vi "Test NI DAQ API.vi"() -> ()   [LabVIEW 2020]
doc: "NI DAQ API Tester."
uses:
  Support/Task list.ctl
  AI config parameters--cluster.ctl
  <vilib>/Utility/error.llb/DialogType.ctl
  Support/Continuous aquisition params.ctl
  NI DAQ.lvlib
  <resource>/objmgr/daqmx.rc
panel:
  in  "Delete task":bool
  out "Digital data":bool[](array[boolean])
  out "Analog data":dbl[](array[numeric])
  in  "Stop continuous acquisition":bool
  in  "N samples":i32
  in  "Acquisition type":enum16{"Single", "Multiple"}(ring)=enum."Multiple"
  in  "Start continous acquisition":bool
  out "DevSerialNum":u32
  out "Connection valid?":bool
  in  "Validate connection":bool
  in  "Sleep HL":bool
  in  "Task list":T1=enum."DO task"
  in  "Timeout":i32=100
  in  "Wake up HL":bool
  in  "Task list 2":T1 caption="Task to get"
  out "DAQmx Task":refnum<k21>
  in  "Get task ref":bool
  in  "Task to stop/delete":T2(ring)
  in  "Tab Control":enum32{"DO", "DI", "AI", "AO"}(tab)
  in  "Create DO task":bool
  in  "Write DO":bool
  in  "Samples":enum16{"Single", "Multiple"}(ring)
  in  "Data":bool[](array[boolean])
  in  "Create DI channel":bool
  in  "Samples 2":enum16{"Single", "Multiple"}(ring) caption="Samples"
  in  "Read DI":bool
  out "Data read":bool[](array[boolean])
  in  "Create AI channel":bool
  in  "Config params":T3={"Terminal configuration"=-1, "min value"=-5.0, "max value"=5.0} {"max value" format="%0.2f"; "min value" format="%0.2f"; "Terminal configuration" items=["Default"=-1, "RSE"=10083, "NRSE"=10078, "Differential"=10106, "Pseudodifferential"=12529]}
  in  "Read AI":bool
  in  "Samples 3":enum16{"Single", "Multiple"}(ring) caption="Samples"
  out "AI Data":dbl[](array[numeric])
  in  "Create AO channel":bool
  in  "Config params 2":T3={"Terminal configuration"=-1, "min value"=-5.0, "max value"=5.0} caption="Config params" {"max value" format="%0.2f"; "min value" format="%0.2f"; "Terminal configuration" items=["Default"=-1, "RSE"=10083, "NRSE"=10078, "Differential"=10106, "Pseudodifferential"=12529]}
  in  "Write AO":bool
  in  "Value(s)":dbl[](array[numeric])
  in  "Samples 4":enum16{"Single", "Multiple"}(ring) caption="Samples"
  in  "Stop task":bool
  in  "Start task":bool
  in  "Channel name":string
  in  "Physical channel(s)":string
  out "Available channels":i32(listbox)
  in  "Get channel list":bool
  in  "Set device ID":bool
  in  "Avilable devices":u16(ring) items=["Dev1"]
  in  "Show Diagram on Init":bool
  in  "Run as Singleton?":bool
  in  "Show Block Diagram":bool
  in  "Refresh Modules":bool
  out "Active Modules":string[](array[string])
  in  "Stop Module":bool
  in  "Select Module":i32(ring)=-1 caption="Select Module\nTo send Request to" items=["All"=-1]
  in  "Run New Module":bool
  in  "Hide Module Panel":bool
  in  "Show Module Panel":bool
  out "Status":string
  # "This VI tests the API for the Module."
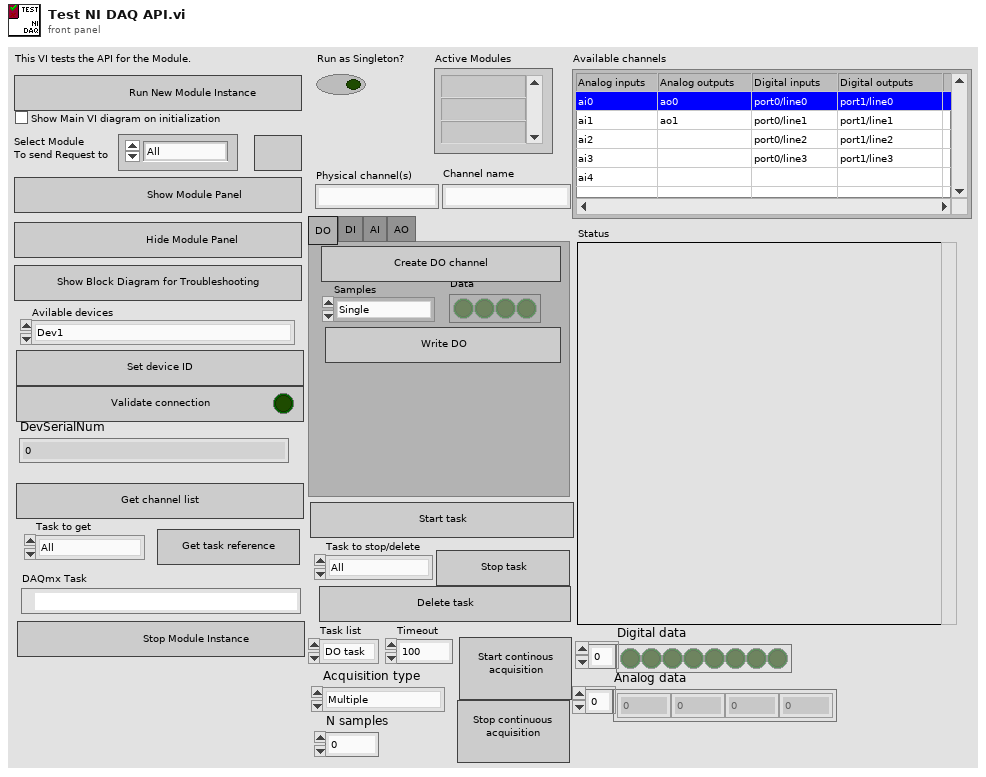
[diagram p1: front panel]
types:
  T1 = typedef "NI DAQ.lvlib/Task list.ctl" = enum16{"All", "DO task", "DI task", "AO task", "AI task"}
  T2 = enum16{"All", "DO task", "DI task", "AO task", "AI task"}
  T3 = typedef "NI DAQ.lvlib/AI config parameters--cluster.ctl" = cluster{"Terminal configuration":i32, "min value":dbl, "max value":dbl}
  T4 = typedef "NI DAQ.lvlib/Broadcast Events--cluster.ctl" = cluster{"Module Did Init":refnum<user-event>, "Status Updated":refnum<user-event>, "Error Reported":refnum<user-event>, "Module Did Stop":refnum<user-event>, "Update Module Execution Status":refnum<user-event>, "Digital data acquired":refnum<user-event>, "Device connected":refnum<user-event>, "Connection failed":refnum<user-event>, "Analog data acquired":refnum<user-event>, "Tasks started":refnum<user-event>}
  T5 = typedef "NI DAQ.lvlib/Continuous aquisition params.ctl" = cluster{"Module ID":i32, "Task list":T1, "Timeout":i32, "Acq type":enum16{"Single", "Multiple"}, "Data in":variant, "DAQmx Task":refnum<k21>, "N samples":i32}
  T6 = typedef "DialogType.ctl" = u16
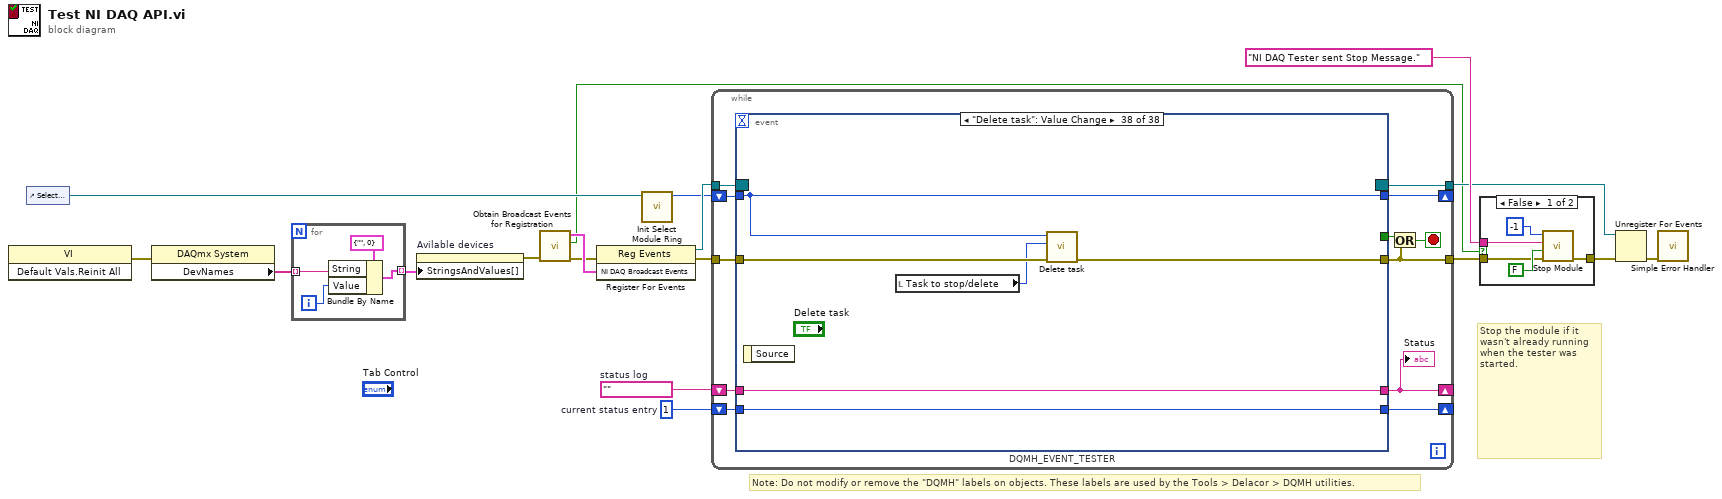
[diagram p0: block diagram]
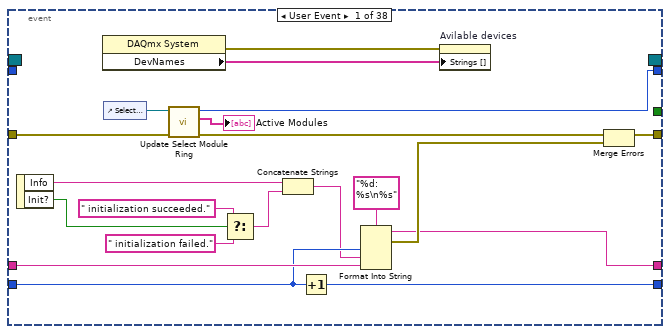
[diagram p3: hidden frame]
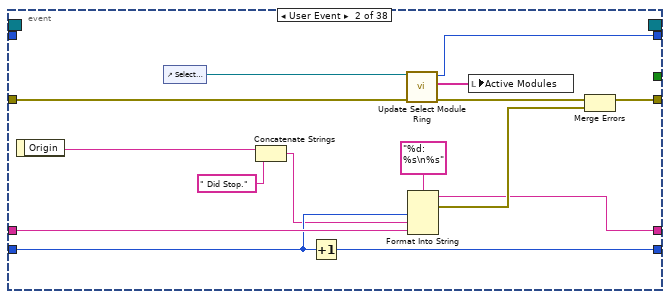
[diagram p4: hidden frame]
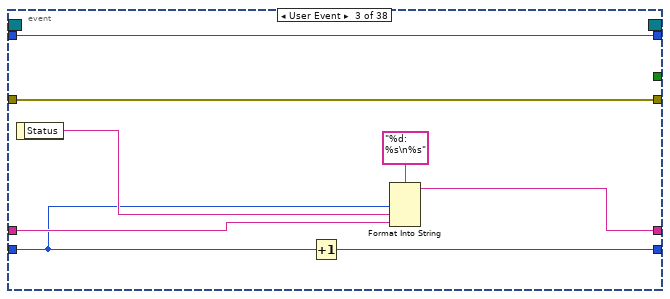
[diagram p5: hidden frame]
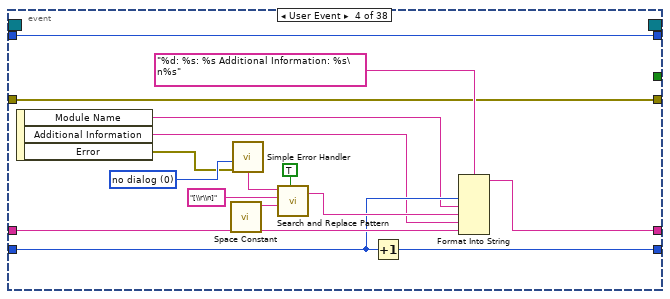
[diagram p6: hidden frame]
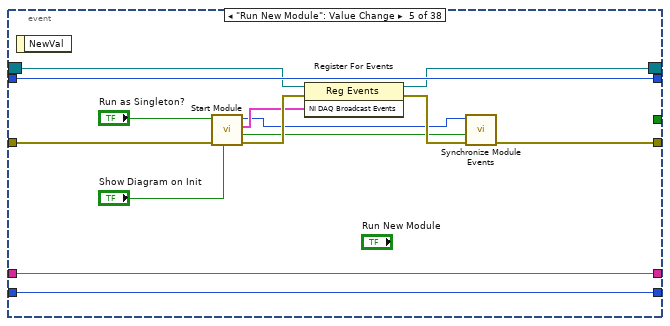
[diagram p7: hidden frame]
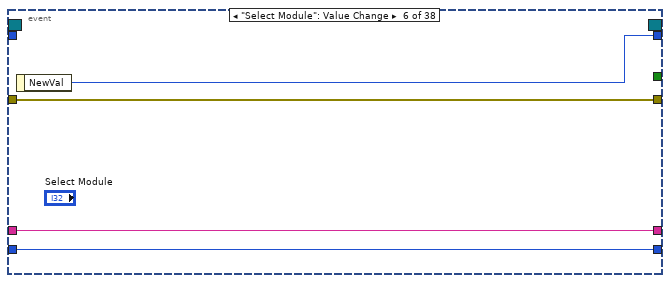
[diagram p8: hidden frame]
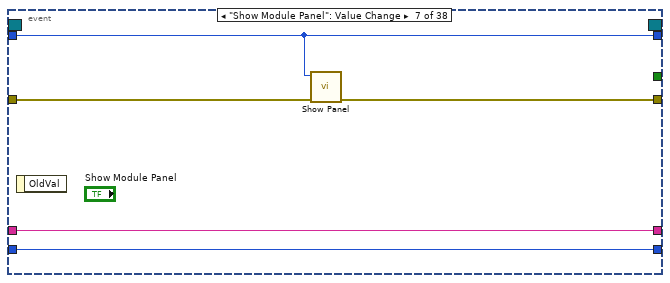
[diagram p9: hidden frame]
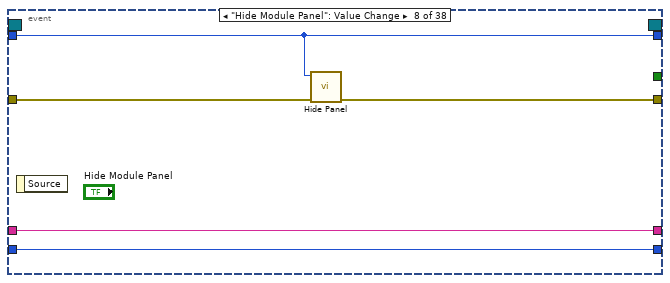
[diagram p10: hidden frame]
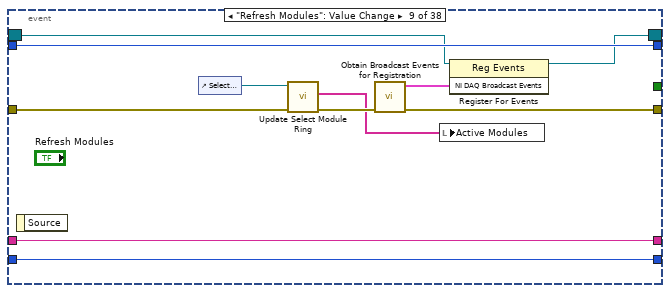
[diagram p11: hidden frame]
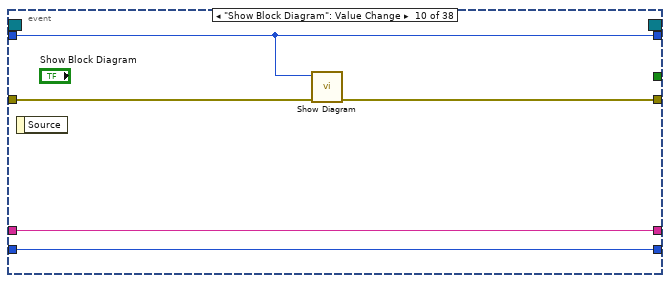
[diagram p12: hidden frame]
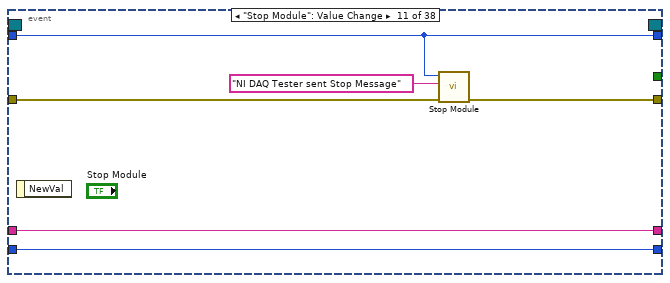
[diagram p13: hidden frame]
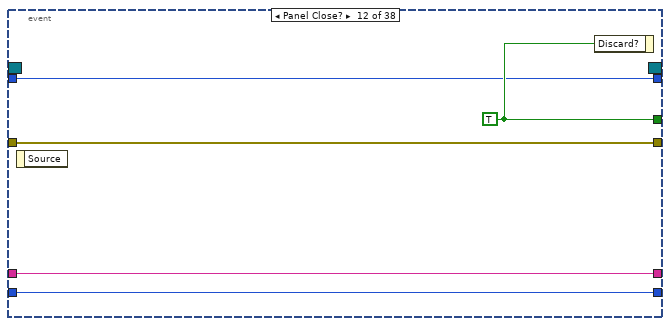
[diagram p14: hidden frame]
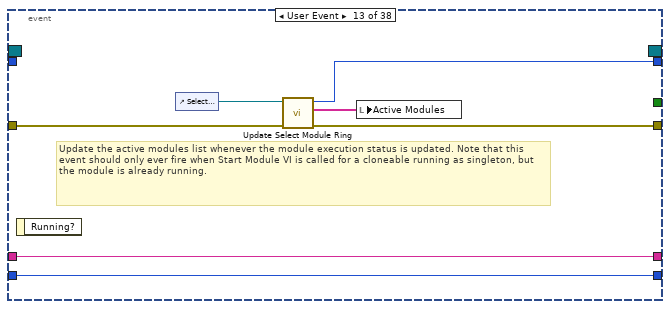
[diagram p15: hidden frame]
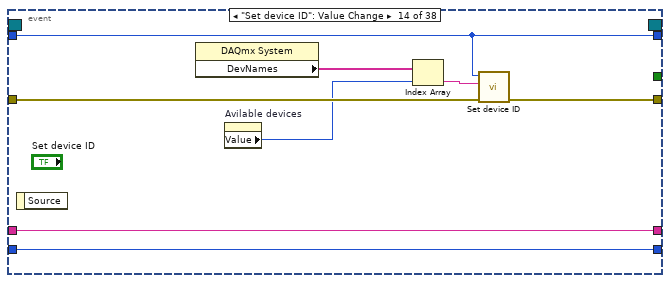
[diagram p16: hidden frame]
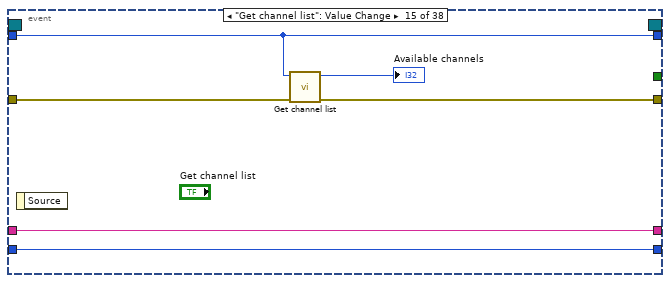
[diagram p17: hidden frame]
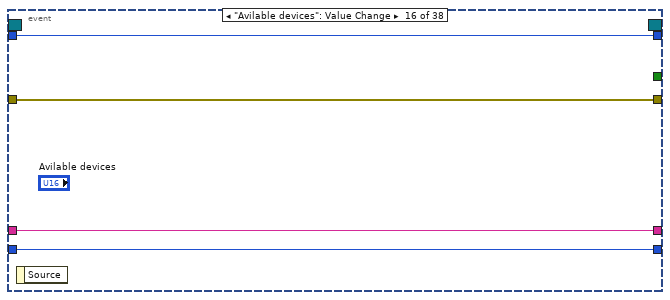
[diagram p18: hidden frame]
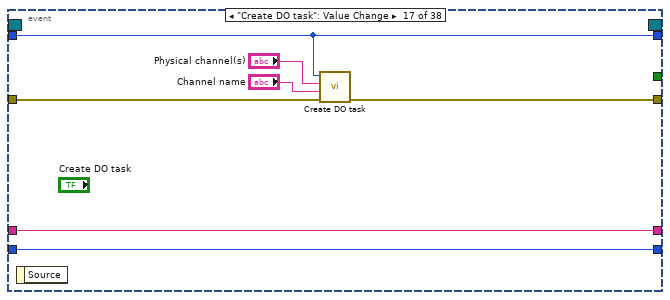
[diagram p19: hidden frame]
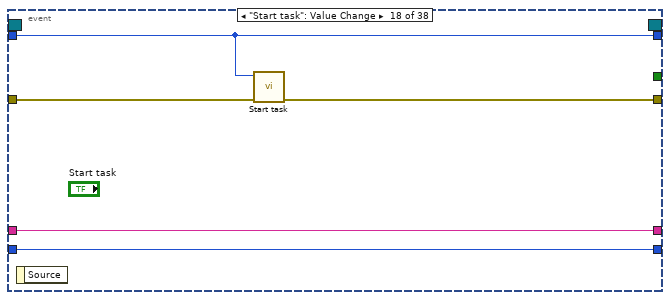
[diagram p20: hidden frame]
diagram:
  w15 = 1  # current status entry
  w16 = ""  # status log
  # "Stop the module if it wasn't already running when the tester was started."
  # "Note: Do not modify or remove the \"DQMH\" labels on objects. These labels are used by the Tools > Delacor > DQMH utilities."
  n1 = invoke class="VI" method="Default Vals.Reinit All"() -> (error out=w4:errorcluster)  [unwired: 3 in, 2 out]
  n2 = control-ref of="Select Module"() -> (w13:refnum<vi>)
  n3 = property class="DAQmx System"(error in=w4) -> ("DevNames"=w3:tag[])  [unwired: 1 in, 2 out]
  n4 = for {
    tunnel: w3 -> [w21] mode=indexing
    tunnel: [w19] -> w2 mode=indexing
    i -> [w20]
    n5 = Bundle By Name(cluster=cluster{"String":string, "Value":u16} {"String"="", "Value"=0} ("Cluster"), "String"=w21, "Value"=w20) -> (w19:cluster{"String":string, "Value":u16})
  }
  n6 = property on="Avilable devices" class="Ring (strict)"("StringsAndValues[]"=w2) -> (error out=w1:errorcluster)  [unwired: 2 in, 1 out]
  n7 = call "Obtain Broadcast Events for Registration.vi"("error in"=w1) -> ("error out"=w8:errorcluster, "Already running?"=w7:bool, "NI DAQ Broadcast Events"=w12:T4)  [unwired: 8 in]
  n8 = register-events(error in=w8, w12) -> (reference out=w18:refnum<event-registration>, error out=w11:errorcluster)  [unwired: 1 in]
  n9 = call "Init Select Module Ring.vi"("Select Module Ring Ref"=w13) -> ("Value for All Modules"=w14:i32)  [unwired: 8 in, 2 out]
  n10 = while {
    tunnel: w18 -> [w34]
    tunnel: [w23] -> w6
    tunnel: w11 -> [w32]
    shift-right: [w28] -> _
    shift-left: w16 -> [w30]
    shift-right: [w29] -> _
    shift-left: w15 -> [w31]
    shift-right: [w25] -> _
    shift-left: w14 -> [w26]
    tunnel: [w24] -> w9
    stop <- w27 stop-if-true
    n11 = event "DQMH_EVENT_TESTER" shown="[37] \"Delete task\": Value Change" {
      selector: w34 -> [_ _ _ _ w101 _ _ _ w127 _ _ _ _ _ _ _ _ _ _ _ _ _ _ _ _ _ _ _ _ _ _ _ _ _ _ _ _ _]
      dyn-events: [_ _ _ _ w100 _ _ _ w126 _ _ _ _ _ _ _ _ _ _ _ _ _ _ _ _ _ _ _ _ _ _ _ _ _ _ _ _ _] -> w24
      timeout: _ -> [_ _ _ _ _ _ _ _ _ _ _ _ _ _ _ _ _ _ _ _ _ _ _ _ _ _ _ _ _ _ _ _ _ _ _ _ _ _]
      tunnel: [_ _ _ _ _ _ _ _ _ _ _ w148 _ _ _ _ _ _ _ _ _ _ _ _ _ _ _ _ _ _ _ _ _ _ _ _ _ _] -> w33
      tunnel: [w45 w61 w77 w81 w99 w111 w115 w120 w123 w134 w139 w147 w151 w160 w166 w173 w177 w182 w188 w195 w202 w209 w216 w230 w234 w248 w253 w260 w268 w275 w281 w295 w306 w312 w317 w331 w341 w343] -> w23
      tunnel: w32 -> [w46 w63 w77 w81 w102 w111 w116 w121 w128 w137 w140 w147 w152 w163 w169 w173 w180 w185 w191 w198 w205 w212 w219 w229 w237 w248 w256 w263 w271 w278 w284 w295 w306 w315 w320 w331 w341 w347]
      tunnel: w31 -> [w51 w66 w70 w84 w104 w109 w113 w118 w131 w135 w142 w145 w154 w161 w167 w171 w178 w183 w189 w196 w203 w210 w217 w231 w235 w244 w254 w261 w269 w276 w282 w291 w302 w313 w318 w327 w337 w345]
      tunnel: w30 -> [w52 w67 w73 w85 w105 w110 w114 w119 w132 w136 w143 w146 w155 w162 w168 w172 w179 w184 w190 w197 w204 w211 w218 w232 w236 w246 w255 w262 w270 w277 w283 w293 w304 w314 w319 w329 w339 w346]
      tunnel: [w49 w64 w74 w83 w105 w110 w114 w119 w132 w136 w143 w146 w155 w162 w168 w172 w179 w184 w190 w197 w204 w211 w218 w232 w236 w245 w255 w262 w270 w277 w283 w292 w303 w314 w319 w328 w338 w346] -> w28
      tunnel: [w50 w65 w76 w82 w104 w109 w113 w118 w131 w135 w142 w145 w154 w161 w167 w171 w178 w183 w189 w196 w203 w210 w217 w231 w235 w243 w254 w261 w269 w276 w282 w290 w301 w313 w318 w326 w336 w345] -> w29
      tunnel: w26 -> [_ _ w71 w93 w103 _ w112 w117 w130 w133 w141 w144 _ w159 w165 w170 w176 w181 w187 w194 w201 w208 w215 w227 w233 w247 w252 w259 w267 w274 w280 w294 w305 w311 w316 w330 w340 w344]
      tunnel: [w37 w58 w71 w93 w103 w108 w112 w117 w130 w133 w141 w144 w150 w159 w165 w170 w176 w181 w187 w194 w201 w208 w215 w227 w233 w247 w252 w259 w267 w274 w280 w294 w305 w311 w316 w330 w340 w344] -> w25
      event User Event {
        n12 = event-data() -> ("Info"=w48:string, "Init?"=w40:bool)  [unwired: 1 in]
        n13 = property class="DAQmx System"() -> (error out=w36:errorcluster, "DevNames"=w35:tag[])  [unwired: 2 in, 1 out]
        n14 = control-ref of="Select Module"() -> (w44:refnum<vi>)
        n15 = call "Update Select Module Ring.vi"("error in (no error)"=w46, "Select Module Ring Ref"=w44) -> ("error out"=w38:errorcluster, "Active Modules (Array)"=→"Active Modules":string[], "New Module Ring Value"=w37:i32)  [unwired: 7 in]
        n16 = Select(t=" initialization succeeded.", s=w40, f=" initialization failed.") -> (s? t:f=w39:string)
        n17 = Concatenate Strings(w48, w39) -> (w47:string)
        n18 = Increment(x=w51) -> (x+1=w50:i32)
        n19 = Format Into String(format string="%d: %s\n%s", w51, w47, w52) -> (resulting string=w49:string, error out=w54:errorcluster)  [unwired: 2 in]
        n20 = property on="Avilable devices" class="Ring (strict)"(error in=w36, "Strings []"=w35) -> ()  [unwired: 1 in, 2 out]
        n21 = Merge Errors(w38, w54) -> (w45:errorcluster)
      }
      event User Event {
        n22 = event-data() -> ("Origin"=w56:string)  [unwired: 1 in]
        n23 = control-ref of="Select Module"() -> (w60:refnum<vi>)
        n24 = Concatenate Strings(w56, " Did Stop.") -> (w55:string)
        n25 = Increment(x=w66) -> (x+1=w65:i32)
        n26 = call "Update Select Module Ring.vi"("error in (no error)"=w63, "Select Module Ring Ref"=w60) -> ("error out"=w62:errorcluster, "Active Modules (Array)"=w59:string[], "New Module Ring Value"=w58:i32)  [unwired: 7 in]
        n27 = Format Into String(format string="%d: %s\n%s", w66, w55, w67) -> (resulting string=w64:string, error out=w69:errorcluster)  [unwired: 2 in]
        n28 = local write "Active Modules"(w59) -> ()
        n29 = Merge Errors(w62, w69) -> (w61:errorcluster)
      }
      event User Event {
        n30 = event-data() -> ("Status"=w72:string)  [unwired: 1 in]
        n31 = Increment(x=w70) -> (x+1=w76:i32)
        n32 = Format Into String(format string="%d: %s\n%s", w70, w72, w73) -> (resulting string=w74:string)  [unwired: 2 in, 1 out]
      }
      event User Event {
        w86 = T6 0 items=["no dialog", "OK message", "continue or stop message", "OK message + warnings", "continue/stop + warnings"] ("type of dialog (OK msg:1)")
        n33 = event-data() -> ("Module Name"=w80:string, "Additional Information"=w79:string, "Error"=w78:errorcluster)  [unwired: 1 in]
        n34 = call <vilib>:"Space Constant.vi"() -> ("String"=w90:string)
        n35 = call <vilib>:"Simple Error Handler.vi"("type of dialog (OK msg:1)"=w86, "error in (no error)"=w78) -> ("message"=w87:string)  [unwired: 3 in, 4 out]
        n36 = call <vilib>:"Search and Replace Pattern.vi"("string"=w87, "regular expression (\"\")"="[\\r\\n]" ("regular expression (\"\")"), "replace string (\"\")"=w90, "replace all? (F)"=TRUE ("replace all CR/LF with spaces")) -> ("result string"=w88:string)  [unwired: 1 in, 1 out]
        n37 = Increment(x=w84) -> (x+1=w82:i32)
        n38 = Format Into String(format string="%d: %s: %s Additional Information: %s\n%s", w84, w80, w88, w79, w85) -> (resulting string=w83:string)  [unwired: 2 in, 1 out]
      }
      event "Run New Module": Value Change {
        n39 = event-data() -> ()  [unwired: 1 in, 1 out]
        n40 = call "Start Module.vi"("Show Main VI Diagram on Init (F)"="Show Diagram on Init", "error in"=w102, "Run as Singleton? (F)"="Run as Singleton?") -> ("error out"=w106:errorcluster, "Wait for Event Sync?"=w98:bool, "NI DAQ Broadcast Events"=w97:T4, "Module ID"=w94:i32)  [unwired: 5 in]
        n41 = register-events(reference=w101, error in=w106, w97) -> (reference out=w100:refnum<event-registration>, error out=w107:errorcluster)
        n42 = call "Synchronize Module Events.vi"("error in"=w107, "Wait for Event Sync?"=w98, "Module ID in"=w94) -> ("error out"=w99:errorcluster)  [unwired: 7 in, 1 out]
      }
      event "Select Module": Value Change {
        n43 = event-data() -> ("NewVal"=w108:i32)  [unwired: 1 in]
      }
      event "Show Module Panel": Value Change {
        n44 = event-data() -> ()  [unwired: 1 in, 1 out]
        n45 = call "Show Panel.vi"("error in (no error)"=w116, "Module ID"=w112) -> ("error out"=w115:errorcluster)  [unwired: 9 in]
      }
      event "Hide Module Panel": Value Change {
        n46 = event-data() -> ()  [unwired: 1 in, 1 out]
        n47 = call "Hide Panel.vi"("error in (no error)"=w121, "Module ID"=w117) -> ("error out"=w120:errorcluster)  [unwired: 9 in]
      }
      event "Refresh Modules": Value Change {
        n48 = event-data() -> ()  [unwired: 1 in, 1 out]
        n49 = control-ref of="Select Module"() -> (w129:refnum<vi>)
        n50 = call "Update Select Module Ring.vi"("error in (no error)"=w128, "Select Module Ring Ref"=w129) -> ("error out"=w124:errorcluster, "Active Modules (Array)"=w122:string[])  [unwired: 7 in, 1 out]
        n51 = call "Obtain Broadcast Events for Registration.vi"("error in"=w124) -> ("error out"=w123:errorcluster, "NI DAQ Broadcast Events"=w125:T4)  [unwired: 8 in, 1 out]
        n52 = local write "Active Modules"(w122) -> ()
        n53 = register-events(reference=w127, w125) -> (reference out=w126:refnum<event-registration>)  [unwired: 1 in, 1 out]
      }
      event "Show Block Diagram": Value Change {
        n54 = event-data() -> ()  [unwired: 1 in, 1 out]
        n55 = call "Show Diagram.vi"("error in (no error)"=w137, "Module ID"=w133) -> ("error out"=w134:errorcluster)  [unwired: 9 in]
      }
      event "Stop Module": Value Change {
        n56 = event-data() -> ()  [unwired: 1 in, 1 out]
        n57 = call "Stop Module.vi"("error in"=w140, "Origin"="NI DAQ Tester sent Stop Message", "Module ID"=w141) -> ("error out"=w139:errorcluster)  [unwired: 8 in]
      }
      event Panel Close? {
        w148 = TRUE ("Discard?")
        n58 = event-data() -> ()  [unwired: 1 in, 1 out]
        n59 = event-data("Discard?"=w148) -> ()  [unwired: 1 in, 1 out]
      }
      event User Event {
        # "Update the active modules list whenever the module execution status is updated. Note that this event should only ever fire when Start Module VI is called for a cloneable running as singleton, but the module is already running."
        n60 = event-data() -> ()  [unwired: 1 in, 1 out]
        n61 = control-ref of="Select Module"() -> (w153:refnum<vi>)
        n62 = call "Update Select Module Ring.vi"("error in (no error)"=w152, "Select Module Ring Ref"=w153) -> ("error out"=w151:errorcluster, "Active Modules (Array)"=w149:string[], "New Module Ring Value"=w150:i32)  [unwired: 7 in]
        n63 = local write "Active Modules"(w149) -> ()
      }
      event "Set device ID": Value Change {
        n64 = event-data() -> ()  [unwired: 1 in, 1 out]
        n65 = property class="DAQmx System"() -> ("DevNames"=w156:tag[])  [unwired: 2 in, 2 out]
        n66 = property on="Avilable devices" class="Ring (strict)"() -> ("Value"=w158:u16)  [unwired: 2 in, 2 out]
        n67 = Index Array(array=w156, index=w158) -> (element=w157:tag)
        n68 = call "Set device ID.vi"("error in"=w163, "Device ID"=w157, "Module ID"=w159) -> ("error out"=w160:errorcluster)  [unwired: 8 in]
      }
      event "Get channel list": Value Change {
        n69 = event-data() -> ()  [unwired: 1 in, 1 out]
        n70 = call "Get channel list.vi"("error in"=w169, "Module ID"=w165) -> ("error out"=w166:errorcluster, "Available channels"=→"Available channels":i32)  [unwired: 7 in, 1 out]
      }
      event "Avilable devices": Value Change {
        n71 = event-data() -> ()  [unwired: 1 in, 1 out]
      }
      event "Create DO task": Value Change {
        n72 = event-data() -> ()  [unwired: 1 in, 1 out]
        n73 = call "Create DO task.vi"("error in"=w180, "Channel name"="Channel name", "lines"="Physical channel(s)", "Module ID"=w176) -> ("error out"=w177:errorcluster)  [unwired: 5 in, 2 out]
      }
      event "Start task": Value Change {
        n74 = event-data() -> ()  [unwired: 1 in, 1 out]
        n75 = call "Start task.vi"("error in"=w185, "Module ID"=w181) -> ("error out"=w182:errorcluster)  [unwired: 9 in]
      }
      event "Stop task": Value Change {
        n76 = event-data() -> ()  [unwired: 1 in, 1 out]
        n77 = call "Stop task.vi"("error in"=w191, "Task list"="Task to stop/delete", "Module ID"=w187) -> ("error out"=w188:errorcluster)  [unwired: 8 in]
      }
      event "Write DO": Value Change {
        n78 = event-data() -> ()  [unwired: 1 in, 1 out]
        n79 = call "Write DO.vi"("error in"=w198, "Samples"="Samples", "Data"="Data", "Module ID"=w194) -> ("error out"=w195:errorcluster)  [unwired: 7 in]
      }
      event "Create DI channel": Value Change {
        n80 = event-data() -> ()  [unwired: 1 in, 1 out]
        n81 = local read "Physical channel(s)"() -> (w200:string)
        n82 = local read "Channel name"() -> (w199:string)
        n83 = call "Create DI channel.vi"("error in"=w205, "Channel name"=w199, "Physical channel"=w200, "Module ID"=w201) -> ("error out"=w202:errorcluster)  [unwired: 7 in]
      }
      event "Read DI": Value Change {
        n84 = event-data() -> ()  [unwired: 1 in, 1 out]
        n85 = call "Read DI.vi"("error in"=w212, "Samples"="Samples 2", "Module ID"=w208) -> ("error out"=w209:errorcluster, "Data"=→"Data read":bool[])  [unwired: 6 in, 1 out]
      }
      event "Get task ref": Value Change {
        n86 = event-data() -> ()  [unwired: 1 in, 1 out]
        n87 = call "Get task ref.vi"("error in"=w219, "Task list"="Task list 2", "Module ID"=w215) -> ("error out"=w216:errorcluster, "DAQmx Task"=→"DAQmx Task":refnum<k21>)  [unwired: 6 in, 1 out]
      }
      event "Wake up HL": Value Change {
        n88 = event-data() -> ()  [unwired: 1 in, 1 out]
        n89 = call "Get task ref.vi"("error in"=w229, "Task list"="Task list", "Module ID"=w227) -> ("error out"=w228:errorcluster)  [unwired: 6 in, 2 out]
        n90 = local read "Data"() -> (w224:bool[])
        n91 = Bundle By Name(cluster=T5 {"Module ID"=0, "Task list"=enum."All", "Timeout"=0, "Acq type"=enum."Single", "Data in"=variant, "DAQmx Task"="", "N samples"=0} ("Acquisition data"), "Task list"="Task list", "Timeout"="Timeout", "Acq type"=enum16{"Single", "Multiple"}."Multiple" ("Samples"), "Data in"=w224) -> (w220:T5)
        n92 = call "Wake up HL.vi"("wait for reply (T)"=FALSE, "error in"=w228, "Acquisition data"=w220, "Module ID"=w227) -> ("error out"=w230:errorcluster)  [unwired: 5 in, 2 out]
      }
      event "Sleep HL": Value Change {
        n93 = event-data() -> ()  [unwired: 1 in, 1 out]
        n94 = call "Sleep HL.vi"("error in"=w237, "Module ID"=w233) -> ("error out"=w234:errorcluster)  [unwired: 9 in]
      }
      event User Event {
        n95 = event-data() -> ("Data"=→"Digital data":bool[])  [unwired: 1 in]
        n96 = Format Into String(format string="Response Received - %s", "Data acquired." ("input 1")) -> (resulting string=w240:string)  [unwired: 2 in, 1 out]
        n97 = Increment(x=w244) -> (x+1=w243:i32)
        n98 = Format Into String(format string="%d: %s\n%s", w244, w240, w246) -> (resulting string=w245:string)  [unwired: 2 in, 1 out]
      }
      event "Create AI channel": Value Change {
        n99 = event-data() -> ()  [unwired: 1 in, 1 out]
        n100 = local read "Physical channel(s)"() -> (w251:string)
        n101 = local read "Channel name"() -> (w250:string)
        n102 = call "Create AI channel.vi"("Config params"="Config params", "error in"=w256, "Channel name"=w250, "Physical channel"=w251, "Module ID"=w252) -> ("error out"=w253:errorcluster)  [unwired: 6 in]
      }
      event "Read AI": Value Change {
        n103 = event-data() -> ()  [unwired: 1 in, 1 out]
        n104 = call "Read AI.vi"("error in"=w263, "Samples"="Samples 3", "Module ID"=w259) -> ("error out"=w260:errorcluster, "Data"=→"AI Data":dbl[])  [unwired: 6 in, 1 out]
      }
      event "Create AO channel": Value Change {
        n105 = event-data() -> ()  [unwired: 1 in, 1 out]
        n106 = local read "Physical channel(s)"() -> (w266:string)
        n107 = local read "Channel name"() -> (w265:string)
        n108 = call "Create AO channel.vi"("Config params"="Config params 2", "error in"=w271, "Channel name"=w265, "Physical channel"=w266, "Module ID"=w267) -> ("error out"=w268:errorcluster)  [unwired: 6 in]
      }
      event "Write AO": Value Change {
        n109 = event-data() -> ()  [unwired: 1 in, 1 out]
        n110 = call "Write AO.vi"("error in"=w278, "Samples"="Samples 4", "Value(s)"="Value(s)", "Module ID"=w274) -> ("error out"=w275:errorcluster)  [unwired: 7 in]
      }
      event "Validate connection": Value Change {
        n111 = event-data() -> ()  [unwired: 1 in, 1 out]
        n112 = call "Validate connection.vi"("error in"=w284, "Module ID"=w280) -> ("error out"=w281:errorcluster, "DevSerialNum"=→"DevSerialNum":u32)  [unwired: 7 in, 1 out]
      }
      event User Event {
        n113 = event-data() -> ("Connected?"=→"Connection valid?":bool)  [unwired: 1 in]
        n114 = Format Into String(format string="Response Received - %s", "Device connected" ("input 1")) -> (resulting string=w287:string)  [unwired: 2 in, 1 out]
        n115 = Increment(x=w291) -> (x+1=w290:i32)
        n116 = Format Into String(format string="%d: %s\n%s", w291, w287, w293) -> (resulting string=w292:string)  [unwired: 2 in, 1 out]
      }
      event User Event {
        n117 = event-data() -> ("Connected?"=w297:bool)  [unwired: 1 in]
        n118 = local write "Connection valid?"(w297) -> ()
        n119 = Format Into String(format string="Response Received - %s", "Connection failed." ("input 1")) -> (resulting string=w298:string)  [unwired: 2 in, 1 out]
        n120 = Increment(x=w302) -> (x+1=w301:i32)
        n121 = Format Into String(format string="%d: %s\n%s", w302, w298, w304) -> (resulting string=w303:string)  [unwired: 2 in, 1 out]
      }
      event "Start continous acquisition": Value Change {
        n122 = event-data() -> ()  [unwired: 1 in, 1 out]
        n123 = local read "Task list"() -> (w309:T1)
        n124 = local read "Timeout"() -> (w308:i32)
        n125 = call "Start continous acquisition.vi"("N samples"="N samples", "Samples"="Acquisition type", "error in"=w315, "Timeout"=w308, "Task list"=w309, "Module ID"=w311) -> ("error out"=w312:errorcluster)  [unwired: 5 in]
      }
      event "Stop continuous acquisition": Value Change {
        n126 = event-data() -> ()  [unwired: 1 in, 1 out]
        n127 = call "Stop continuous acquisition.vi"("error in"=w320, "Module ID"=w316) -> ("error out"=w317:errorcluster)  [unwired: 9 in]
      }
      event User Event {
        n128 = event-data() -> ("Data"=→"Analog data":dbl[])  [unwired: 1 in]
        n129 = Format Into String(format string="Response Received - %s", "Analog data acquired." ("input 1")) -> (resulting string=w323:string)  [unwired: 2 in, 1 out]
        n130 = Increment(x=w327) -> (x+1=w326:i32)
        n131 = Format Into String(format string="%d: %s\n%s", w327, w323, w329) -> (resulting string=w328:string)  [unwired: 2 in, 1 out]
      }
      event User Event {
        n132 = event-data() -> ()  [unwired: 1 in, 5 out]
        n133 = Format Into String(format string="Response Received - %s", "Tasks successfuly started." ("input 1")) -> (resulting string=w333:string)  [unwired: 2 in, 1 out]
        n134 = Increment(x=w337) -> (x+1=w336:i32)
        n135 = Format Into String(format string="%d: %s\n%s", w337, w333, w339) -> (resulting string=w338:string)  [unwired: 2 in, 1 out]
      }
      event "Delete task": Value Change {
        n136 = event-data() -> ()  [unwired: 1 in, 1 out]
        n137 = local read "Task to stop/delete"() -> (w342:T2)
        n138 = call "Delete task.vi"("error in"=w347, "Task to stop/delete"=w342, "Module ID"=w344) -> ("error out"=w343:errorcluster)  [unwired: 8 in]
      }
    }
    "Status" <- w28
    n139 = Or(x=w33, y=w23) -> (x .or. y?=w27:bool)
  }
  n140 = case shown="False" w7 {
    tunnel: [w352 w353] -> w17
    tunnel: "NI DAQ Tester sent Stop Message." ("Origin") -> [w351 _]
    tunnel: w6 -> [w348 w353]
    frame False {
      n141 = call "Stop Module.vi"("error in"=w348, "Wait for Module to stop? (F)"=FALSE ("Wait for Module to stop?"), "Origin"=w351, "Module ID"=-1 ("Stop all")) -> ("error out"=w352:errorcluster)  [unwired: 7 in]
    }
    frame True {
    }
  }
  n142 = Unregister For Events(event registration refnum=w9, error in=w17) -> (error out=w5:errorcluster)
  n143 = call <vilib>:"Simple Error Handler.vi"("error in (no error)"=w5) -> ()  [unwired: 4 in, 5 out]
